vi "AlliGator Get IRF from Decay v2.vi"(8 "error in (no error)":errorcluster, 11 "Selected Plot Info":T1={"Multiplot XY Graph"=refnum, "Mouse Coordinates"={"Horizontal"=0, "Vertical"=0}, "Plot Index"=-1}) -> (0 "Error Out":errorcluster, 1 "Message":string, 3 "Extracted IRF":cluster{"t Array":dbl[], "IRF Array":dbl[]})   [LabVIEW 2021, in "AlliGator IRF.lvlib"]
doc: "Extract IRF by deconvolution with a single-exponential decay with the provided time constant."
uses:
  Graphs/XY Graph/XY Graph Selected Plot Info.ctl
  Graphs/XY Graph/XY Graph Refnum.ctl
  <vilib>/Utility/miscctls.llb/LVPoint32TypeDef.ctl
  Settings/AlliGator Settings List.ctl
  Fits/IRF(X)PSED/IRF(X)PSED Fixed Parameters v3.ctl
  Fits/IRF(X)PSED/IRF(X)PSED Extraction Options.ctl
  Fits/IRF(X)PSED/Fourier Series Smoothing Option.ctl
  Fits/IRF(X)PSED/Fourier Series Truncation.ctl
  Fits/IRF(X)PSED/IRF Extraction Method.ctl
  Fits/Fit Plot Request Information.ctl
  <vilib>/Utility/miscctls.llb/LVPointDoubleTypeDef.ctl
  Fits/Fit Models.ctl
  Graphs/XY Graph/XY Graph Add Single Plot with Name.vi
  AlliGator IRF.lvlib
  Graphs/XY Graph/XY Graph Add-Ons.lvlib
  Settings/AlliGator Settings.lvlib
  Fits/Fits.lvlib
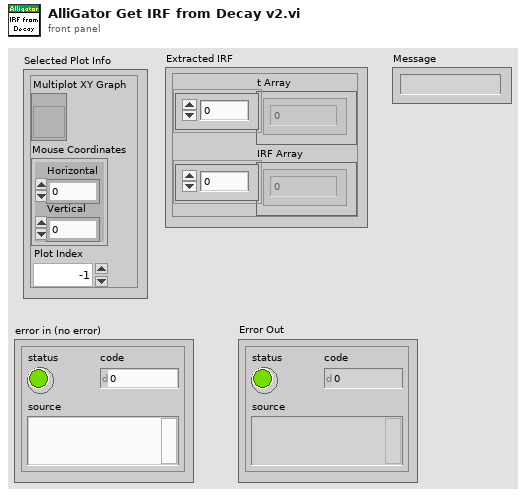
[diagram p1: front panel]
types:
  T1 = typedef "XY Graph Add-Ons.lvlib/XY Graph Selected Plot Info.ctl" = cluster{"Multiplot XY Graph":T2, "Mouse Coordinates":T3, "Plot Index":i32}
  T2 = typedef "XY Graph Add-Ons.lvlib/XY Graph Refnum.ctl" = refnum<vi>
  T3 = typedef "LVPoint32TypeDef.ctl" = cluster{"Horizontal":i32, "Vertical":i32}
  T4 = typedef "Fits.lvlib/IRF Extraction Method.ctl" = enum16{"Direct", "Topless", "Toeplitz"}
  T5 = typedef "Fits.lvlib/Fit Plot Request Information.ctl" = cluster{"XY Graph Ref":refnum<vi>, "Mouse Coordinates":T6, "Fit Model":T7, "Plot Index":i32}
  T6 = typedef "LVPointDoubleTypeDef.ctl" = cluster{"X":dbl, "Y":dbl}
  T7 = typedef "Fits.lvlib/Fit Models.ctl" = enum16{"Select a Fit Model...", "           Single Peak", "Gaussian", "Asymmetric Gaussian", "Lorentzian", "Asymmetric Lorentzian", "Gaussian/Lorentzian", "Lorentzian/Gaussian", "           Double Peak", "Two Gaussians", "Two Asymmetric Gaussians", "Two H-Connected Gaussians", "Two T-Connected Gaussians", "Two H-Connected Asymmetric Gaussians", "Two T-Connected Asymmetric Gaussians", "           Triple Peak", "Three Gaussians", "Three Asymmetric Gaussians", "              Decays", "1-Exponential", "IRF*PSED", "2-Exponentials", "            Power Law", "Power Law", "Power Law with Offset", "               ACF", "2D Gaussian ACF", "2D Gaussian + Blinking ACF", "2D Gaussian + Flow ACF", "3D Gaussian ACF", "3D Gaussian + Blinking ACF", "             Multiplot", "2D Gaussian ACF & 2D Gaussian + Flow ACF"}
  T8 = typedef "Fits.lvlib/IRF(X)PSED Extraction Options.ctl" = cluster{"Time Constant for IRF Extraction":dbl[unit], "IRF Order":i32, "Fourier Series Smoothing":T9, "Noise Threshold":dbl, "Smoothing Width":dbl, "Fourier Series Truncation":T10, "Truncation Order":i32, "Save Power Spectrum":bool, "Smoothing":bool, "Smoothing Parameter":dbl, "Smoothing Order":u32, "Method":T4}
  T9 = typedef "Fits.lvlib/Fourier Series Smoothing Option.ctl" = enum16{"None", "Lanczos Factors", "Fejer Summation"}
  T10 = typedef "Fits.lvlib/Fourier Series Truncation.ctl" = enum16{"Automatic", "Fixed"}
  T11 = typedef "Fits.lvlib/IRF(X)PSED Fixed Parameters v3.ctl" = cluster{"order":i32, "T":dbl, "Time Constant Array":dbl[], "{S_k, C_k, phi_k, e_k} arrays":cluster{"S_k Array":dbl[], "C_k Array":dbl[], "phi_k Array":dbl[], "e_k Array":dbl[]}, "IRF Extraction Options":T8}
  T12 = typedef "AlliGator Settings.lvlib/AlliGator Settings List.ctl" = enum16{"GUI:Visible Settings Tab", "GUI:Last Run Version", "Source Image:Use Image Histogram for Contrast", "Source Image:Low Count Pixels Rejection Options", "Source Image:High Count Pixels Rejection Options", "Source Image:Use Image Brightness", "Source Image:Blend Overlay with Image Background", "Source Image:Use Fixed ROI Diameter", "Source Image:ROI Diameter", "Source Image:ROI Center Color", "Source Image:Peak Threshold", "Source Image:Intensity Threshold", "Source Image:Image Binning Options", "Source Image:Image Smoothing Options", "Source Image:Image Histogram Active", "Source Image:Invert Binary Mask", "Source Image:Hot Pixel Removal", "Source Image:Overlay Analyzed ROI Center", "Source Image:Auto-Adjust Contrast", "Source Image:Histogram Lower Percentile", "Source Image:Histogram Upper Percentile", "Source Image:Save Source Image", "Source Image:Scale Bar Options", "Source Image:Image Resolution (Pixel Size)", "Source Image:Flatfield Correction", "Source Image:Show Dead Left Columns Correction", "Source Image:Dead Left Columns Correction", "Source Image:Image Pre-Processing Operations Order", "Source Image:Overlay ROI Median", "Source Image:Median Overlay Color", "Data Information:Gate Width", "Data Information:Nanotime Gate Separation", "Data Information:Macrotime Gate Separation", "Data Information:Gate Step", "Data Information:# Gates", "Data Information:Gate Image Exposure", "Data Information:Gate Image Integration", "Data Information:Gates to Skip", "Data Information:Gates to Keep", "Data Information:Define Gates to", "Data Information:Channel Name", "Data Information:Available Channel Names", "Data Information:Channel Arithmetic", "Data Information:Background File Subtraction", "Data Information:Background File", "Data Information:Background Scaling Factor", "Data Information:Background Pile-up Correction", "Data Information:Background Pixel Well Capacity", "Data Information:Laser Period", "Data Information:SYNC Period", "Data Information:Pile-up Correction", "Data Information:Pixel Well Capacity", "Data Information:Dataset Scaling Factor", "Fluorescence Decay_Decay Pre-Processing:Reverse Gates", "Fluorescence Decay_Decay Pre-Processing:Verbose Decay Pre-Processing", "Fluorescence Decay_Decay Pre-Processing:Use Decay Pre-Processing", "Fluorescence Decay_Decay Pre-Processing:Background Subtraction", "Fluorescence Decay_Decay Pre-Processing:Background Definition Range", "Fluorescence Decay_Decay Pre-Processing:Baseline Subtraction Method", "Fluorescence Decay_Decay Pre-Processing:Decay Pre-Processing Operations Order", "Fluorescence Decay_Decay Pre-Processing:Smoothing Parameter", "Fluorescence Decay_Decay Pre-Processing:Shift Decay", "Fluorescence Decay_Decay Pre-Processing:Decay Shift Parameters", "Fluorescence Decay_Decay Pre-Processing:Fold Decay", "Fluorescence Decay_Decay Pre-Processing:# Folds", "Fluorescence Decay_Decay Pre-Processing:1-Normalize Decay", "Fluorescence Decay_Decay Pre-Processing:[0-1]-Normalize Decay", "Fluorescence Decay_Decay Pre-Processing:Smoothen Decay", "Fluorescence Decay_Decay Pre-Processing:Extrapolate Decay", "Fluorescence Decay_Decay Pre-Processing:Use Periodicity", "Fluorescence Decay_Decay Pre-Processing:Use Cursors", "Fluorescence Decay_Decay Pre-Processing:Tail Fraction", "Fluorescence Decay_Decay Pre-Processing:Head Fraction", "Fluorescence Decay_Decay Pre-Processing:Additional Points", "Fluorescence Decay_Decay Pre-Processing:Straighten Decay", "Fluorescence Decay_Decay Pre-Processing:Constant Background", "Fluorescence Decay_Decay Pre-Processing:Pixel-Normalize Decay", "Fluorescence Decay_Advanced Analysis:Extract IRF instead of Decay", "Fluorescence Decay_Advanced Analysis:IRF Extraction Options", "Fluorescence Decay_Advanced Analysis:IRF Optimization Options", "Fluorescence Decay_Advanced Analysis:Square Pulse Options", "Fluorescence Decay_Advanced Analysis:IRF Order", "Fluorescence Decay_Advanced Analysis:IRF Time Constants", "Fluorescence Decay_Advanced Analysis:Wavelet Analysis Options", "Fluorescence Decay_Advanced Analysis:Average Lifetime Options", "Fluorescence Decay_Fit Options:Fit Options", "Fluorescence Decay_Fit Options:Use Legacy Fitting Approach", "Fluorescence Decay_Fit Options:Use Data Information Laser Period", "Fluorescence Decay_Fit Parameters:Displayed Fit Parameters", "Fluorescence Decay_Fit Parameters:Fit Parameter Constraints", "Fluorescence Decay_Fit Parameters:Export Tabulated Results", "Fluorescence Decay_Fit Parameters:MLE Baseline Offset Type", "Fluorescence Decay_Fit Parameters:MLE Baseline Offset", "Fluorescence Decay_Fit Parameters:Guess Parameter Names", "Fluorescence Decay_Fit Parameters:Guess Parameter Values", "Fluorescence Decay_Fit Parameters:Guess Parameters Options", "Fluorescence Decay_Fit Parameters:Optimal Offset Selection Criterion", "Fluorescence Decay_Styles:Show Last Decay Only", "Fluorescence Decay_Styles:Decay Graph Color Array", "Fluorescence Decay:Decay Graph Active", "Fluorescence Decay Statistics:Min Peak Value", "Fluorescence Decay Statistics:Reject Low Decay Peak Pixels", "Fluorescence Decay Statistics:Reject High Decay Peak Pixels", "Fluorescence Decay Statistics:Max Peak Value", "Time Traces:Use File Timestamp", "Time Traces:Time Step", "Time Traces:Use Intensity Correction File", "Time Traces:Intensity Correction File", "Phasor Plot:Phasor Plot Smoothing Options", "Phasor Plot:Phasor Plot Size", "Phasor Plot:Phasor Plot Graphics Options", "Phasor Plot:Cumulative Phasor Plot", "Phasor Plot:Use Phasor Brightness", "Phasor Plot:Blend Overlay with Phasor Background", "Phasor Plot:Save Phasor Plot", "Phasor Plot:Show References", "Phasor Plot:Phasor Ratio Decay Range", "Phasor Plot:Exponential Fading", "Phasor Plot:Phasor Ratio Reference Colors", "Phasor Plot:Reference Radius", "Phasor Plot:Show Color Map Vertices", "Phasor Plot:Phasor Plot Active", "Phasor Plot:Phasor Ratio Color Map Type", "Phasor Plot:Phasor Ratio Color Map", "Phasor Plot:Phasor Ratio Display Range", "Phasor Plot:Selected Image ROI(s)", "Phasor Plot:All Image ROIs", "Phasor Plot:Selected Phasor Plot ROI(s)", "Phasor Plot:All Phasor Plot ROIs", "Phasor Plot:Phasor Ratio Color-Coded Quantity", "Phasor Plot:Store Phasor Harmonics", "Phasor Plot:Draw Reference Segment", "Phasor Plot:User-Defined Quantity", "Phasor Plot:Color Scale High Color", "Phasor Plot:Color Scale Low Color", "Phasor Plot:Intensity-weighted Phasor Plot", "Phasor Graph:Phasor Frequency", "Phasor Graph:Phasor Ratio Type", "Phasor Graph:Pixel-level Phasor Computation", "Phasor Graph:Save Phasor Graph", "Phasor Graph:Phasor Graph Active", "Phasor Graph:Phasor SDV Options", "Phasor Graph:Intensity-weighted Phasor Graph", "Phasor Graph:Define Shortest Lifetime as", "Phasor Calibration:Use Backup Calibration if needed", "Phasor Calibration:Backup Calibration Type", "Phasor Calibration:Calibration Type", "Phasor Calibration:Calibration Lifetime", "Phasor Calibration:Calibration Map Algorithm", "Single-Exponential Phasor Locus (SEPL):Gate Parameters", "Single-Exponential Phasor Locus (SEPL):User-defined Gate", "Single-Exponential Phasor Locus (SEPL):User-defined IRF", "Single-Exponential Phasor Locus (SEPL):Phasor Parameters", "Single-Exponential Phasor Locus (SEPL):Decay & IRF Parameters", "Single-Exponential Phasor Locus (SEPL):Display Parameters", "Lifetime Analysis:Decay Analysis Parameters", "Lifetime Analysis:Lifetime Map Active", "Plugins:Python Settings", "Miscellaneous:Verbose Mode", "Miscellaneous:Beep after Script", "Miscellaneous:Saved Image File Format", "Miscellaneous:Exported Gate Image Settings", "Miscellaneous:Include Loading in Timing", "Miscellaneous:Verbose Settings Mode", "Miscellaneous:Histogram Options", "Miscellaneous:Beep on Error", "Miscellaneous:# Logical Processors Used", "Miscellaneous:ROI Description Max Characters", "Miscellaneous:Verbose Error Mode", "Miscellaneous:Transparent Mask Color"}
  T13 = typedef "XY Graph Add-Ons.lvlib/XY Graph Plot Data.ctl" = cluster{"X Array":dbl[], "Y Array":dbl[]}
  T14 = cluster{"t Array (dup)":dbl[], "IRF Array":dbl[]}
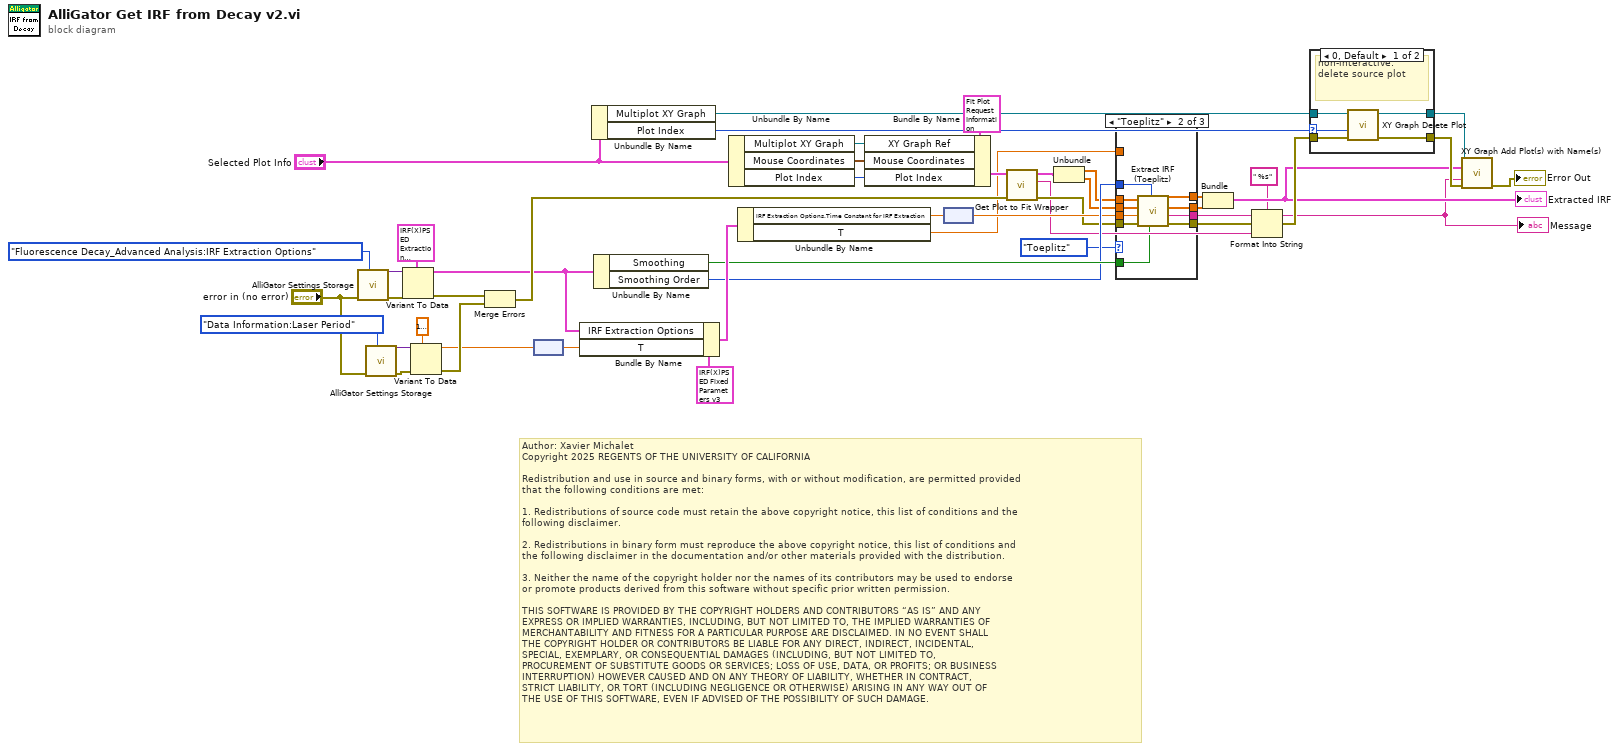
[diagram p0: block diagram]
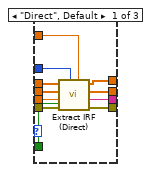
[diagram p3: hidden frame]
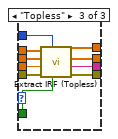
[diagram p4: hidden frame]
diagram:
  # "Author: Xavier Michalet\nCopyright 2025 REGENTS OF THE UNIVERSITY OF CALIFORNIA\n\nRedistribution and use in source and binary forms, with or without modification, are permitted provided\nthat the following conditions are met:\n\n1. Redistributions of source code must retain the above copyright notice, this list of conditions and the\nfollowing disclaimer.\n\n2. Redistributions in binary form must reproduce the above copyright notice, this list of conditions and\nthe following disclaimer in the documentation and/or other materials provided with the distribution.\n\n3. Neither the name of the copyright holder nor the names of its contributors may be used to endorse \nor promote products derived from this software without specific prior written permission.\n\nTHIS SOFTWARE IS PROVIDED BY THE COPYRIGHT HOLDERS AND CONTRIBUTORS “AS IS” AND ANY \nEXPRESS OR IMPLIED WARRANTIES, INCLUDING, BUT NOT LIMITED TO, THE IMPLIED WARRANTIES OF\nMERCHANTABILITY AND FITNESS FOR A PARTICULAR PURPOSE ARE DISCLAIMED. IN NO EVENT SHALL\nTHE COPYRIGHT HOLDER OR CONTRIBUTORS BE LIABLE FOR ANY DIRECT, INDIRECT, INCIDENTAL, \nSPECIAL, EXEMPLARY, OR CONSEQUENTIAL DAMAGES (INCLUDING, BUT NOT LIMITED TO, \nPROCUREMENT OF SUBSTITUTE GOODS OR SERVICES; LOSS OF USE, DATA, OR PROFITS; OR BUSINESS\nINTERRUPTION) HOWEVER CAUSED AND ON ANY THEORY OF LIABILITY, WHETHER IN CONTRACT, \nSTRICT LIABILITY, OR TORT (INCLUDING NEGLIGENCE OR OTHERWISE) ARISING IN ANY WAY OUT OF\nTHE USE OF THIS SOFTWARE, EVEN IF ADVISED OF THE POSSIBILITY OF SUCH DAMAGE."
  n1 = call "AlliGator Settings Storage.vi"("AlliGator Settings List"=AlliGator_Settings_List."Fluorescence Decay_Advanced Analysis:IRF Extraction Options", "Error In"="error in (no error)") -> ("Error Out"=w45:errorcluster, "Variant Data out"=w46:variant)  [unwired: 8 in]
  n2 = call "AlliGator Settings Storage.vi"("AlliGator Settings List"=AlliGator_Settings_List."Data Information:Laser Period", "Error In"="error in (no error)") -> ("Error Out"=w40:errorcluster, "Variant Data out"=w42:variant)  [unwired: 8 in]
  n3 = Variant To Data(error in=w45, type=T8 {"Time Constant for IRF Extraction"=4.08e-09, "IRF Order"=132, "Fourier Series Smoothing"=enum."Fejer Summation", "Noise Threshold"=0.1, "Smoothing Width"=0.1, "Fourier Series Truncation"=enum."Automatic", "Truncation Order"=0, "Save Power Spectrum"=FALSE, "Smoothing"=FALSE, "Smoothing Parameter"=0.0, "Smoothing Order"=1, "Method"=enum."Direct"} ("IRF Extraction Options"), Variant=w46) -> (data=w28:T8, error out=w44:errorcluster)
  n4 = Variant To Data(error in=w40, type=dbl[unit] 1e-09 ("Time Constant"), Variant=w42) -> (data=w38:dbl[unit], error out=w39:errorcluster)
  n5 = Merge Errors(w44, w39) -> (w36:errorcluster)
  n6 = node(w38) -> (w32:dbl)
  n7 = Bundle By Name(cluster=T11 {"order"=0, "T"=0.0, "Time Constant Array"=[], "{S_k, C_k, phi_k, e_k} arrays"={"S_k Array"=[], "C_k Array"=[], "phi_k Array"=[], "e_k Array"=[]}, "IRF Extraction Options"={"Time Constant for IRF Extraction"=1e-18, "IRF Order"=0, "Fourier Series Smoothing"=enum."None", "Noise Threshold"=0.0, "Smoothing Width"=0.0, "Fourier Series Truncation"=enum."Automatic", "Truncation Order"=0, "Save Power Spectrum"=FALSE, "Smoothing"=FALSE, "Smoothing Parameter"=0.0, "Smoothing Order"=1, "Method"=enum."Direct"}} ("IRF*PSED Fixed Parameters"), "IRF Extraction Options"=w28, "T"=w32) -> (w30:T11)
  n8 = Unbundle By Name("Selected Plot Info") -> ("Multiplot XY Graph"=w33:T2, "Plot Index"=w34:i32)
  n9 = Unbundle By Name(w28) -> ("Smoothing"=w21:bool, "Smoothing Order"=w20:u32)
  n10 = Unbundle By Name("Selected Plot Info") -> ("Multiplot XY Graph"=w10:T2, "Mouse Coordinates"=w9:T3, "Plot Index"=w8:i32)
  n11 = Unbundle By Name(w30) -> ("IRF Extraction Options.Time Constant for IRF Extraction"=w19:dbl[unit], "T"=w2:dbl)
  n12 = Bundle By Name(cluster=T5 {"XY Graph Ref"=refnum, "Mouse Coordinates"={"X"=0.0, "Y"=0.0}, "Fit Model"=enum."Select a Fit Model...", "Plot Index"=0} ("Fit Plot Information"), "XY Graph Ref"=w10, "Mouse Coordinates"=w9, "Plot Index"=w8) -> (w7:T5)
  n13 = node(w19) -> (w18:dbl)
  n14 = call "Get Plot to Fit Wrapper.vi"("error in (no error)"=w36, "Fit Plot Information"=w7) -> ("error out"=w17:errorcluster, "Plot Name"=w3:string, "Clipped Plot"=w16:T13)  [unwired: 3 in, 4 out]
  n15 = Unbundle(w16) -> ("X Array"=w15:dbl[], "Y Array"=w14:dbl[])
  n16 = case shown="\"Toeplitz\"" IRF_Extraction_Method."Toeplitz" ("Method") {
    tunnel: w18 -> [w56 w68 w76]
    tunnel: w17 -> [w55 w67 w75]
    tunnel: w15 -> [w58 w66 w78]
    tunnel: w14 -> [w57 w65 w77]
    tunnel: [w53 w64 w72] -> w13
    tunnel: [w54 w63 w71] -> w12
    tunnel: [w51 w62 w74] -> w5
    tunnel: [w52 w61 w73] -> w4
    tunnel: w21 -> [w50 w60 w69]
    tunnel: w20 -> [w49 w59 w70]
    tunnel: w2 -> [w48 _ _]
    frame "Direct", Default {
      n17 = call "Extract IRF (Direct).vi"("Period"=w48, "Tail Smoothing (T)"=w50, "Smoothing Order"=w49, "Error In"=w55, "Time Constant"=w56, "Intensity Array"=w57, "t Array"=w58) -> ("Error Out"=w51:errorcluster, "Message"=w52:string, "IRF Array"=w53:dbl[], "t Array (dup)"=w54:dbl[])  [unwired: 1 in]
    }
    frame "Toeplitz" {
      n18 = call "Extract IRF (Toeplitz).vi"("Tail Smoothing (T)"=w60, "Smoothing Order"=w59, "Error In"=w67, "Time Constant"=w68, "Intensity Array"=w65, "t Array"=w66) -> ("Error Out"=w62:errorcluster, "Message"=w61:string, "IRF Array"=w64:dbl[], "t Array (dup)"=w63:dbl[])  [unwired: 2 in]
    }
    frame "Topless" {
      n19 = call "Extract IRF (Topless).vi"("Tail Smoothing (T)"=w69, "Smoothing Order"=w70, "Error In"=w75, "Time Constant"=w76, "Intensity Array"=w77, "t Array"=w78) -> ("Error Out"=w74:errorcluster, "Message"=w73:string, "IRF Array"=w72:dbl[], "t Array (dup)"=w71:dbl[])  [unwired: 2 in]
    }
  }
  n20 = Bundle("t Array (dup)"=w12, "IRF Array"=w13) -> (w24:T14)  [unwired: 1 in]
  "Extracted IRF" <- w24
  n21 = Format Into String(format string=" %s", initial string=w4, error in=w5, w3) -> (resulting string=w23:string, error out=w37:errorcluster)
  "Message" <- w23
  n22 = case shown="0, Default" w34 {
    selector: w34 -> [w80 _]
    tunnel: w37 -> [w83 w85]
    tunnel: [w82 w85] -> w27
    tunnel: w33 -> [w81 w84]
    tunnel: [w79 w84] -> w25
    frame 0, Default {
      # "non-interactive: delete source plot"
      n23 = call "XY Graph Delete Plot.vi"("Error In"=w83, "Plot Index"=w80, "XYGraph Ref"=w81) -> ("Error Out"=w82:errorcluster, "XYGraph Ref"=w79:T2)  [unwired: 5 in, 2 out]
    }
    frame -1 {
      # "interactive: keep source plot"
    }
  }
  n24 = call-poly "XY Graph Add Plot(s) with Name(s).vi"("XYGraph Ref in"=w25, "Plot"=w24, "Plot Name (\"Plot\")"=w23, "error in (no error)"=w27) -> ("error out"=→"Error Out":errorcluster)  [unwired: 8 in, 3 out]
